vi "BPSK_XSRPLoopback.vi"(4 "tx_data":dbl[](array[numeric]), 5 "xsrpip":string, 7 "pcip":string, 8 "error in (no error)":errorcluster caption="错误输入（无错误）", 11 "PathIn":path) -> (0 "error out":errorcluster caption="错误输出", 1 "ERR_CODE":dbl, 3 "PathOut":path, 6 "rxdataIQ":cdb[](array[numeric]))   [LabVIEW 2015]
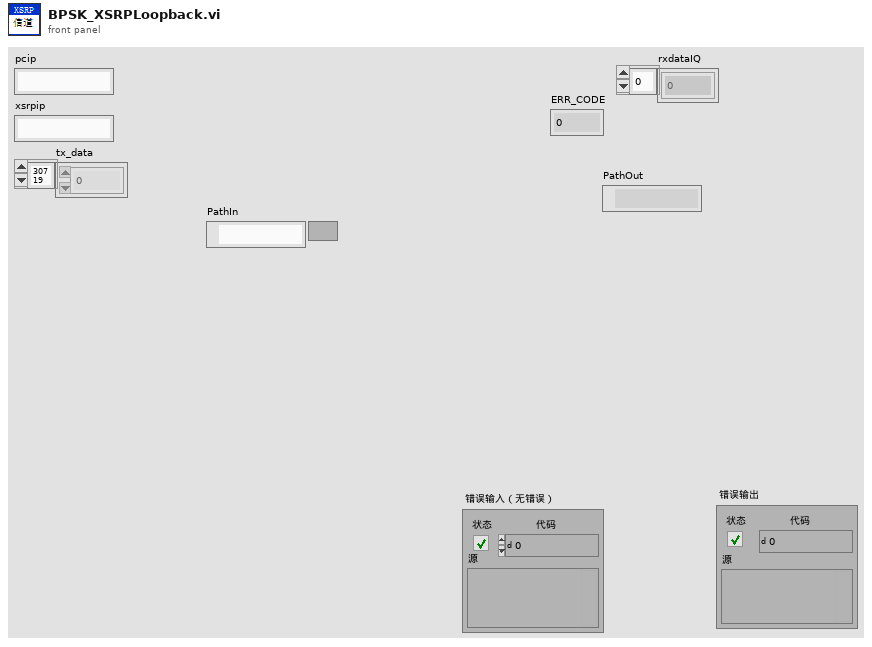
[diagram p1: front panel]
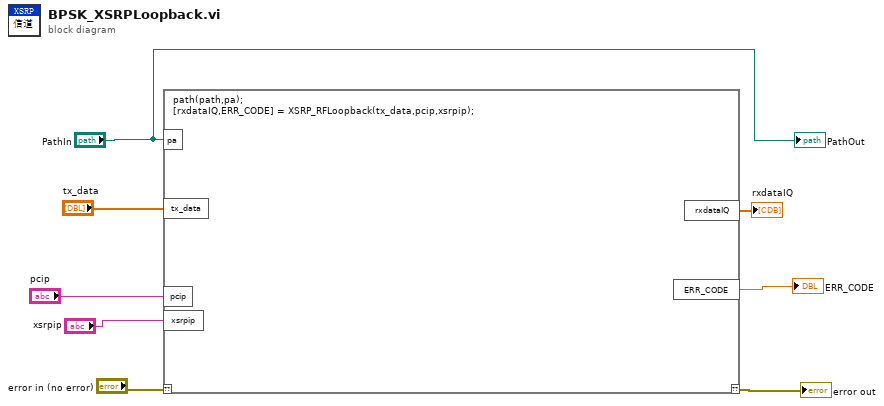
[diagram p0: block diagram]
diagram:
  n1 = script code="path(path,pa);\n[rxdataIQ,ERR_CODE] = XSRP_RFLoopback(tx_data,pcip,xsrpip);"("??"="error in (no error)", "pa"="PathIn", "pcip"="pcip", "xsrpip"="xsrpip", "tx_data"="tx_data") -> ("??"=→"error out":errorcluster, "ERR_CODE"=→"ERR_CODE":dbl, "rxdataIQ"=→"rxdataIQ":cdb[])
  "PathOut" <- "PathIn"
